vi "Get Value Change Trigger.vi"(7 "Trigger Direction":T2, 8 "error in (no error)":errorcluster, 11 "Item Ref in":T3 format="%.0x") -> (0 "error out":errorcluster, 2 "Value Change Trigger":T1, 3 "Item Ref out":T3 format="%.0x")   [LabVIEW 2012, in "Waveform Data Logger Shared.lvlib"]
uses:
  Waveform Data Logger Shared.lvlib
  <vilib>/NI Veristand/Custom Device API/Custom Device Item Ref.ctl
  Types/Trigger Direction.ctl
  Types/Value Change Trigger.ctl
  Globals/Property Strings.vi
  <vilib>/NI Veristand/Custom Device API/Get Item Property (Double).vi
  <vilib>/NI VeriStand/Custom Device API/Custom Device API.lvlib
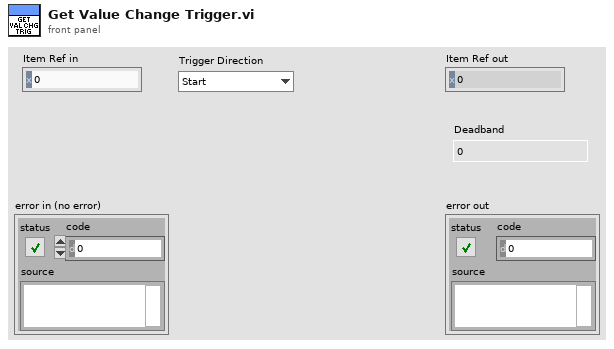
[diagram p1: front panel]
types:
  T1 = typedef "Waveform Data Logger Shared.lvlib/Value Change Trigger.ctl" = cluster{"Deadband":dbl}
  T2 = typedef "Waveform Data Logger Shared.lvlib/Trigger Direction.ctl" = enum16{"Start", "Stop"}
  T3 = typedef "Custom Device API.lvlib/Custom Device Item Ref.ctl" = u64
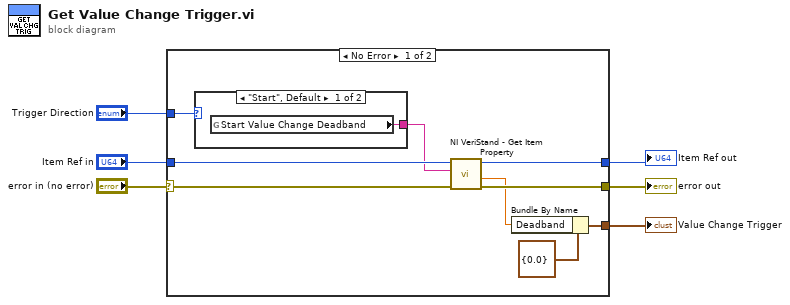
[diagram p0: block diagram]
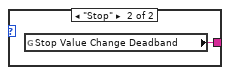
[diagram p2: hidden frame]
diagram:
  n1 = case shown="No Error" "error in (no error)" {
    selector: "error in (no error)" -> [w14 w18]
    tunnel: [w11 w19] -> w6
    tunnel: [w13 w18] -> w5
    tunnel: "Item Ref in" -> [w12 w19]
    tunnel: "Trigger Direction" -> [w15 _]
    tunnel: [w7 _] -> w1
    frame No Error {
      n2 = case shown="\"Start\", Default" w15 {
        tunnel: [w16 w17] -> w10
        frame "Start", Default {
          n3 = global read "Property Strings.vi" "Start Value Change Deadband"() -> (w16:string)
        }
        frame "Stop" {
          n4 = global read "Property Strings.vi" "Stop Value Change Deadband"() -> (w17:string)
        }
      }
      n5 = call-poly <vilib>:"NI VeriStand - Get Item Property.vi"("error in (no error)"=w14, "Property Name"=w10, "Item Ref in"=w12) -> ("error out"=w13:errorcluster, "Value"=w8:dbl, "Item Ref out"=w11:T3)  [unwired: 1 in, 5 out]
      n6 = Bundle By Name(cluster=T1 {"Deadband"=0.0} ("Value Change Trigger"), "Deadband"=w8) -> (w7:T1)
    }
    frame Error {
    }
  }
  "Item Ref out" <- w6
  "error out" <- w5
  "Value Change Trigger" <- w1
